vi "AttributesInfo.vi"() -> ()   [LabVIEW 2014, in "examples.lvlib"]
uses:
  vis/tango_vi.llb/_AttributeAccess_t.ctl
  vis/tango_vi.llb/_AttributeFormat_t.ctl
  vis/tango_vi.llb/_TangoDataType_t.ctl
  vis/tango_vi.llb/_AttributeLevel_t.ctl
  examples.lvlib
  vis/tango_vi.llb/tango.lvlib
panel:
  out "attributes_info":T5(array[cluster])
  in  "device name":string="sys/tg_test/1"
  out "success":bool
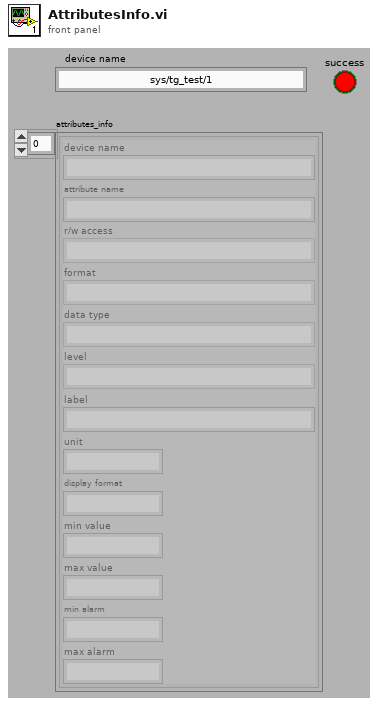
[diagram p1: front panel]
types:
  T1 = typedef "tango.lvlib/_AttributeAccess_t.ctl" = enum16{"READ", "READ_WITH_WRITE", "WRITE", "READ_WRITE", "UNKNOWN_ACCESS_TYPE"}
  T2 = typedef "tango.lvlib/_AttributeFormat_t.ctl" = enum16{"SCALAR", "SPECTRUM", "IMAGE", "UNKNOWN_FORMAT"}
  T3 = typedef "tango.lvlib/_TangoDataType_t.ctl" = enum16{"VOID", "BOOLEAN", "SHORT", "LONG", "FLOAT", "DOUBLE", "USHORT", "ULONG", "STRING", "CHAR_ARRAY", "SHORT_ARRAY", "LONG_ARRAY", "FLOAT_ARRAY", "DOUBLE_ARRAY", "USHORT_ARRAY", "ULONG_ARRAY", "STRING_ARRAY", "LONG_STRING_ARRAY", "DOUBLE_STRING_ARRAY", "STATE", "CONST_STRING", "BOOLEAN_ARRAY", "UCHAR", "LONG64", "ULONG64", "LONG64_ARRAY", "ULONG64_ARRAY", "INT (not supported)", "ENCODED (not supported)", "ENUM", "PIPE_BLOB (not supported)", "STATE_ARRAY", "UNKNOW_DATA_TYPE"}
  T4 = typedef "tango.lvlib/_AttributeLevel_t.ctl" = enum16{"OPERATOR", "EXPERT", "UNKNOWN_LEVEL"}
  T5 = cluster{"device name":string, "attribute name":string, "r/w access":T1, "format":T2, "data type":T3, "level":T4, "label":string, "unit":string, "display format":string, "min value":string, "max value":string, "min alarm":string, "max alarm":string}[]
  T6 = typedef "tango.lvlib/_AttributeInfo_t.ctl" = cluster{"device name":string, "attribute name":string, "r/w access":T1, "format":T2, "data type":T3, "level":T4, "label":string, "unit":string, "display format":string, "min value":string, "max value":string, "min alarm":string, "max alarm":string}
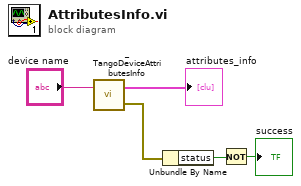
[diagram p0: block diagram]
diagram:
  n1 = call "_TangoDeviceAttributesInfo.vi"("device name"="device name") -> ("error out"=w2:errorcluster, "attributes_info"=→"attributes_info":T6[])  [unwired: 1 in]
  n2 = Unbundle By Name(w2) -> ("status"=w4:bool)
  n3 = Not(x=w4) -> (.not. x?=→"success":bool)
